vi "HCC Get General Configuration Info.vi"(8 "Error In":errorcluster, 11 "General Configuration":path) -> (0 "Error Out":errorcluster, 2 "Network Var Set":u8, 3 "Disable Agilent Collection":bool)   [LabVIEW 2016]
uses:
  <vilib>/Utility/file.llb/Read Delimited Spreadsheet (string).vi
panel:
  out "all rows":string[][](array[string])
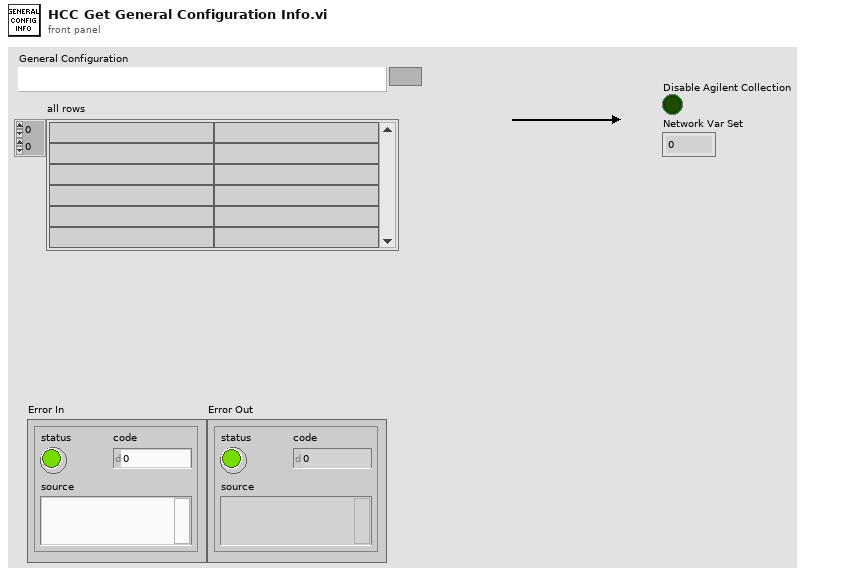
[diagram p1: front panel]
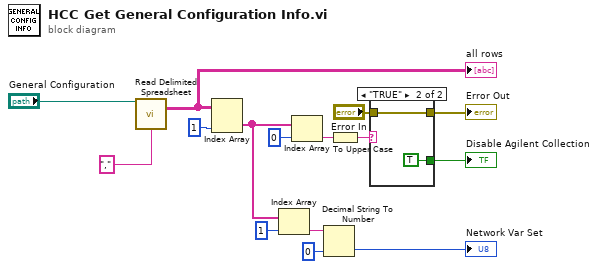
[diagram p0: block diagram]
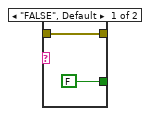
[diagram p2: hidden frame]
diagram:
  n1 = call-poly <vilib>:"Read Delimited Spreadsheet.vi"("file path (dialog if empty)"="General Configuration", "delimiter (\\t)"="," ("delimiter (\\t)")) -> ("all rows"=w6:string[][])  [unwired: 8 in, 5 out]
  "all rows" <- w6
  n2 = Index Array(array=w6, index (col)=1 ("disabled index (col)")) -> (element=w4:string[])  [unwired: 1 in]
  n3 = Index Array(array=w4, index=1) -> (element=w3:string)
  n4 = Index Array(array=w4, index=0) -> (element=w11:string)
  n5 = Decimal String To Number(string=w3, default (0L)=u8 0 ("default (0 I32)")) -> (number=→"Network Var Set":u8)  [unwired: 1 in, 1 out]
  n6 = To Upper Case(1:w11) -> (0:w10:string)
  n7 = case shown="\"TRUE\"" w10 {
    tunnel: [FALSE TRUE] -> w9
    tunnel: "Error In" -> [w16 w18]
    tunnel: [w16 w18] -> w7
    frame "FALSE", Default {
    }
    frame "TRUE" {
    }
  }
  "Error Out" <- w7
  "Disable Agilent Collection" <- w9
